vi "Log Channels to TDMS.vi"(5 "group name in (Group)":string="Group", 6 "Limit(-1)":i32=-1, 7 "NameRule":T2={"FileNameRule"={"Rule"=enum."Fixed File Name", "Path"=path "", "filename"="data.tdms"}, "FileOperation"=enum."create or replace", "byte order (2:little-endian)"=enum."little-endian", "disable buffering? (T)"=TRUE}, 8 "error in (no error)":errorcluster, 9 "TimeChannel(\"\" Empty to Skip)":string="Time", 10 "Array":variant[](array[variant]), 11 "channel names":string[](array[string])) -> (0 "error out":errorcluster, 1 "DataCount":i32, 2 "File":path)   [LabVIEW 2017]
uses:
  _FileName Rule.ctl
  <vilib>/Utility/file.llb/Application Directory.vi
  <userlib>/_OpenG.lib/file/file.llb/Append Path to Root if Relative__ogtk.vi
  <userlib>/_OpenG.lib/file/file.llb/Append Path to Root if Relative - Scalar__ogtk.vi
  <userlib>/_OpenG.lib/file/file.llb/Create Dir if Non-Existant__ogtk.vi
  <userlib>/_MGI/String/MGI Make String Filesafe.vi
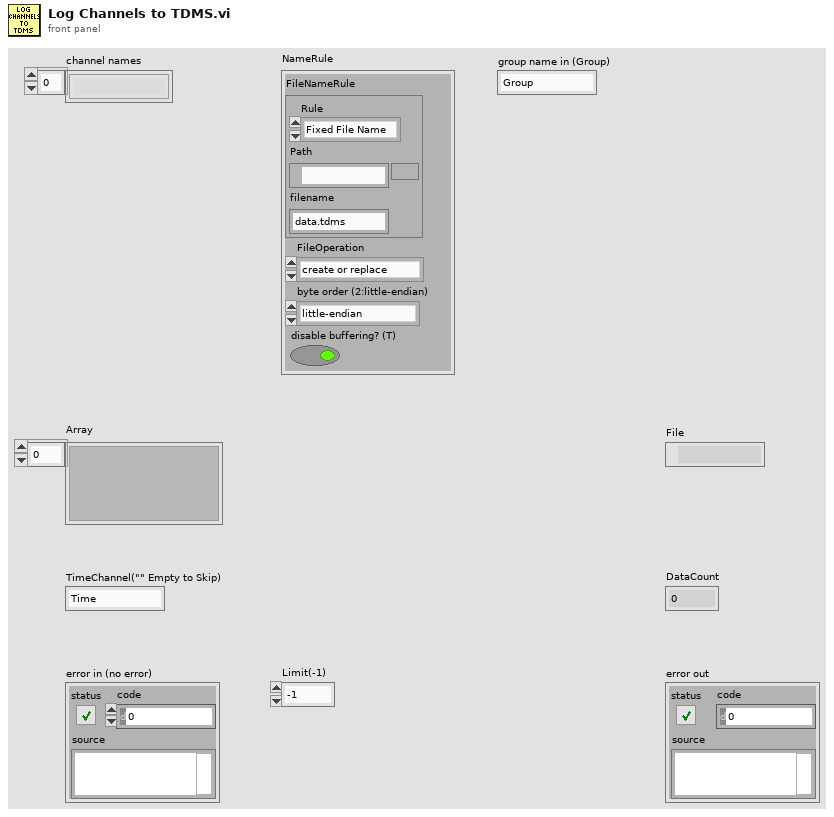
[diagram p1: front panel]
types:
  T1 = typedef "_FileName Rule.ctl" = cluster{"Rule":enum16{"Fixed File Name", "Indexed File Name", "TimeBased File Name"}, "Path":path, "filename":string}
  T2 = cluster{"FileNameRule":T1, "FileOperation":enum16{"open", "open or create", "create or replace", "create", "open (read-only)"}, "byte order (2:little-endian)":enum16{"big-endian, network order", "native, host order", "little-endian"}, "disable buffering? (T)":bool}
  T3 = enum16{"open", "open or create", "create or replace", "create", "open (read-only)"}
  T4 = enum16{"big-endian, network order", "native, host order", "little-endian"}
  T5 = typedef "Type Descriptor Enumeration__ogtk.ctl" = enum8{"<Null>", "I8", "I16", "I32", "I64", "U8", "U16", "U32", "U64", "SGL", "DBL", "EXT", "CSG", "CDB", "CXT", "0x0F", "0x10", "0x11", "0x12", "0x13", "0x14", "Enum U8", "Enum U16", "Enum U32", "Enum U64", "SGL PQ", "DBL PQ", "EXT PQ", "CSG PQ", "CDB PQ", "CXT PQ", "0x1F", "0x20", "Boolean", "0x22", "0x23", "0x24", "0x25", "0x26", "0x27", "0x28", "0x29", "0x2A", "0x2B", "0x2C", "0x2D", "0x2E", "0x2F", "String", "0x31", "Path", "Pict", "0x34", "0x35", "0x36", "DAQ", "0x38", "0x39", "0x3A", "0x3B", "0x3C", "0x3D", "0x3E", "0x3F", "Array", "0x41", "0x42", "0x43", "0x44", "0x45", "0x46", "0x47", "0x48", "0x49", "0x4A", "0x4B", "0x4C", "0x4D", "0x4E", "0x4F", "Cluster", "0x51", "0x52", "Variant", "Waveform", "0x55", "0x56", "0x57", "0x58", "0x59", "0x5A", "0x5B", "0x5C", "0x5D", "0x5E", "0x5F", "0x60", "0x61", "0x62", "0x63", "0x64", "0x65", "0x66", "0x67", "0x68", "0x69", "0x6A", "0x6B", "0x6C", "0x6D", "0x6E", "0x6F", "Refnum"}
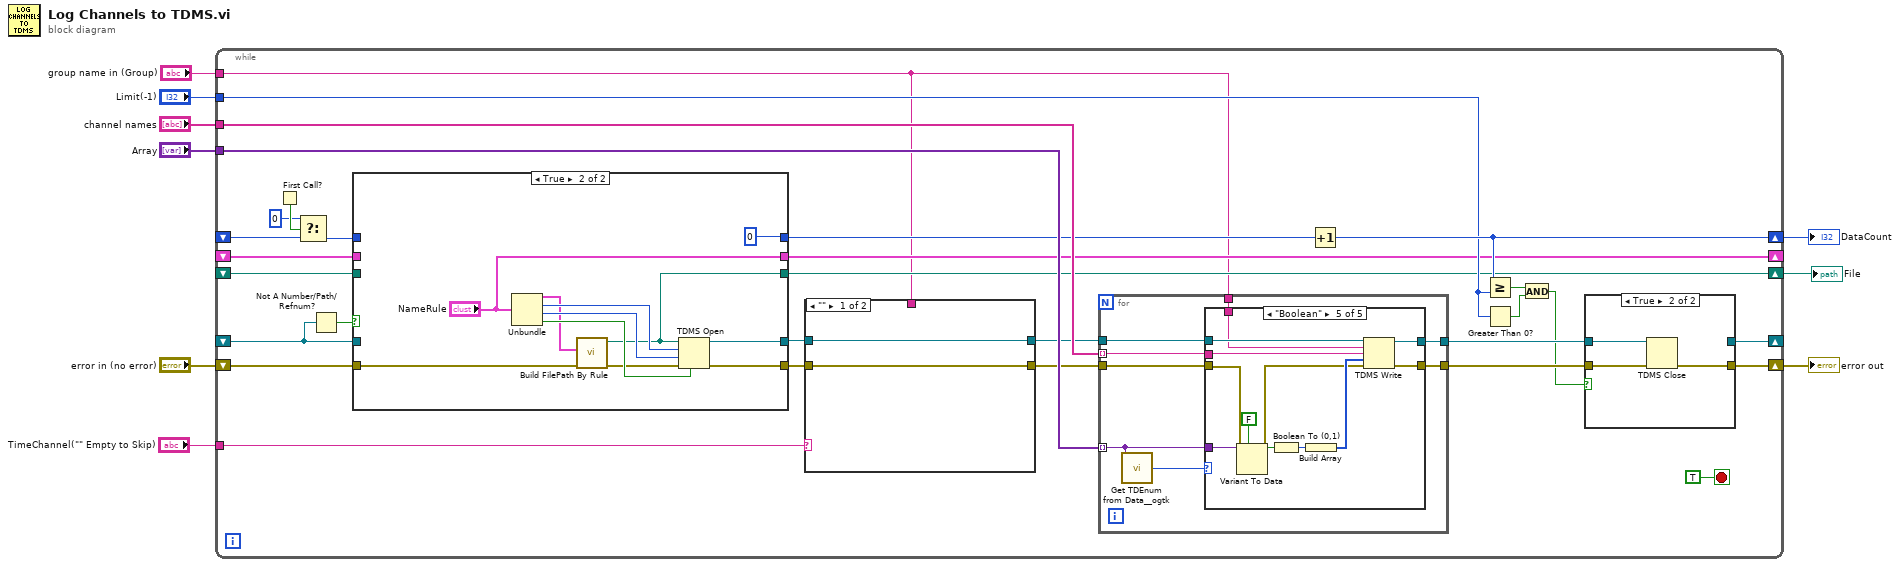
[diagram p0: block diagram]
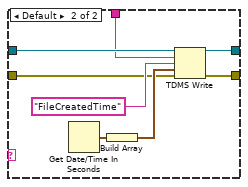
[diagram p2: hidden frame]
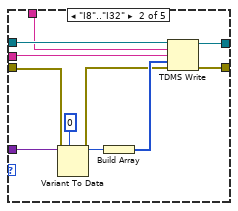
[diagram p4: hidden frame]
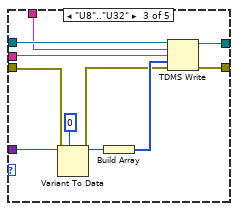
[diagram p5: hidden frame]
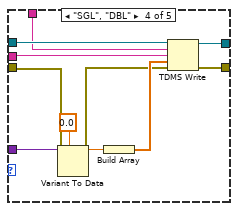
[diagram p6: hidden frame]
diagram:
  n1 = while {
    shift-right: [w39] -> w8
    shift-left: "error in (no error)" -> [w16]
    shift-right: [w38] -> _
    shift-left: _ -> [w36]
    tunnel: "channel names" -> [w34]
    tunnel: "Array" -> [w33]
    shift-right: [w28] -> w4
    shift-left: _ -> [w29]
    tunnel: "Limit(-1)" -> [w26]
    shift-right: [w23] -> w3
    shift-left: _ -> [w22]
    shift-right: [w17] -> _
    shift-left: _ -> [w21]
    tunnel: "TimeChannel(\"\" Empty to Skip)" -> [w11]
    tunnel: "group name in (Group)" -> [w10]
    stop <- TRUE stop-if-true
    n2 = First Call?() -> (First Call?: T/F=w19:bool)
    n3 = Select(t=0, s=w19, f=w29) -> (s? t:f=w20:i32)
    n4 = Not A Number/Path/Refnum?(number/path/refnum=w36) -> (NaN/Path/Refnum?=w37:bool)
    n5 = case shown="True" w37 {
      tunnel: [w114 w117] -> w15
      tunnel: [w113 w116] -> w14
      tunnel: w36 -> [w114 _]
      tunnel: [w112 0] -> w30
      tunnel: w20 -> [w112 _]
      tunnel: [w111 w118] -> w23
      tunnel: w22 -> [w111 _]
      tunnel: w21 -> [w110 _]
      tunnel: [w110 "NameRule"] -> w17
      tunnel: w16 -> [w113 w119]
      frame False {
      }
      frame True {
        n6 = Unbundle("NameRule") -> ("FileNameRule"=w115:T1, "FileOperation"=w121:T3, "byte order (2:little-endian)"=w122:T4, "disable buffering? (T)"=w123:bool)
        n7 = call "Build FilePath By Rule.vi"("error in (no error)"=w119, "FileNameRule"=w115) -> ("error out"=w120:errorcluster, "File"=w118:path)  [unwired: 8 in]
        n8 = TDMS Open(6:w123, 8:w120, 9:w122, 10:w121, 11:w118) -> (0:w116:errorcluster, 3:w117:refnum<k34>)  [unwired: 2 in]
      }
    }
    n9 = case shown="\"\"" w11 {
      tunnel: w15 -> [w41 w46]
      tunnel: w14 -> [w40 w45]
      tunnel: [w41 w44] -> w13
      tunnel: [w40 w43] -> w12
      tunnel: w10 -> [_ w42]
      frame "" {
      }
      frame Default {
        n10 = Get Date/Time In Seconds() -> (seconds since 1Jan1904=w48:timestamp)
        n11 = Build Array(w48) -> (w47:timestamp[])
        n12 = TDMS Write(0:w46, 5:w42, 7:"FileCreatedTime", 9:w47, 11:w45) -> (4:w44:refnum<k34>, 15:w43:errorcluster)  [unwired: 1 in, 2 out]
      }
    }
    n13 = for {
      tunnel: w34 -> [w54] mode=indexing
      tunnel: w33 -> [w57] mode=indexing
      tunnel: w13 -> [w55]
      tunnel: w12 -> [w53]
      tunnel: [w52] -> w32
      tunnel: [w51] -> w31
      tunnel: w10 -> [w50]
      n14 = call <userlib>:"Get TDEnum from Data__ogtk.vi"("Data"=w57) -> ("Type Descriptor Enumeration"=w56:T5)  [unwired: 4 in]
      n15 = case shown="\"Boolean\"" w56 {
        tunnel: w57 -> [_ w68 w79 w90 w102]
        tunnel: w55 -> [w59 w67 w78 w89 w101]
        tunnel: w54 -> [_ w66 w77 w88 w100]
        tunnel: w53 -> [w58 w62 w73 w84 w96]
        tunnel: [w59 w64 w75 w86 w98] -> w52
        tunnel: [w58 w63 w74 w85 w97] -> w51
        tunnel: w50 -> [_ w60 w71 w82 w93]
        frame Default {
        }
        frame "I8".."I32" {
          n16 = Variant To Data(error in=w62, type=0, Variant=w68) -> (data=w69:i32, error out=w61:errorcluster)
          n17 = Build Array(w69) -> (w65:i32[])
          n18 = TDMS Write(0:w67, 5:w60, 7:w66, 9:w65, 11:w61) -> (4:w64:refnum<k34>, 15:w63:errorcluster)  [unwired: 1 in, 2 out]
        }
        frame "U8".."U32" {
          n19 = Variant To Data(error in=w73, type=u32 0, Variant=w79) -> (data=w80:u32, error out=w72:errorcluster)
          n20 = Build Array(w80) -> (w76:u32[])
          n21 = TDMS Write(0:w78, 5:w71, 7:w77, 9:w76, 11:w72) -> (4:w75:refnum<k34>, 15:w74:errorcluster)  [unwired: 1 in, 2 out]
        }
        frame "SGL", "DBL" {
          n22 = Variant To Data(error in=w84, type=0.0, Variant=w90) -> (data=w91:dbl, error out=w83:errorcluster)
          n23 = Build Array(w91) -> (w87:dbl[])
          n24 = TDMS Write(0:w89, 5:w82, 7:w88, 9:w87, 11:w83) -> (4:w86:refnum<k34>, 15:w85:errorcluster)  [unwired: 1 in, 2 out]
        }
        frame "Boolean" {
          n25 = Variant To Data(error in=w96, type=FALSE, Variant=w102) -> (data=w103:bool, error out=w95:errorcluster)
          n26 = Boolean To (0,1)(Boolean=w103) -> (0, 1=w94:i16)
          n27 = Build Array(w94) -> (w99:i16[])
          n28 = TDMS Write(0:w101, 5:w93, 7:w100, 9:w99, 11:w95) -> (4:w98:refnum<k34>, 15:w97:errorcluster)  [unwired: 1 in, 2 out]
        }
      }
    }
    n29 = Increment(x=w30) -> (x+1=w28:i32)
    n30 = Greater Or Equal?(x=w28, y=w26) -> (x >= y?=w27:bool)
    n31 = Greater Than 0?(x=w26) -> (x > 0?=w25:bool)
    n32 = And(x=w27, y=w25) -> (x .and. y?=w24:bool)
    n33 = case shown="True" w24 {
      tunnel: w31 -> [w105 w109]
      tunnel: w32 -> [w106 w108]
      tunnel: [w105 w107] -> w39
      tunnel: [w106 _] -> w38
      frame False {
      }
      frame True {
        n34 = TDMS Close(8:w109, 11:w108) -> (0:w107:errorcluster)  [unwired: 1 out]
      }
    }
  }
  "error out" <- w8
  "DataCount" <- w4
  "File" <- w3
